vi "Write Contents.vi"(8 "Error in":errorcluster caption="Error in (no error)", 10 "Contents":refnum<class "Data Item.lvclass">[](array[class]), 11 "Element Array":refnum<class "Element Array.lvclass">) -> (0 "Error out":errorcluster, 3 "Element Array Out":refnum<class "Element Array.lvclass">)   [LabVIEW 2023, in "VILab.lvlib" / "Element Array.lvclass"]
uses:
  Element Array.lvclass
  Data Item.lvclass
  Attribute.lvclass/Attribute.ctl
  Element Array.lvclass/Element Array.ctl
  Attribute/Create Attribute (Data Item).vi
  Attribute.lvclass
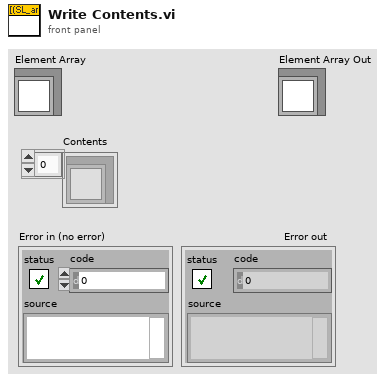
[diagram p1: front panel]
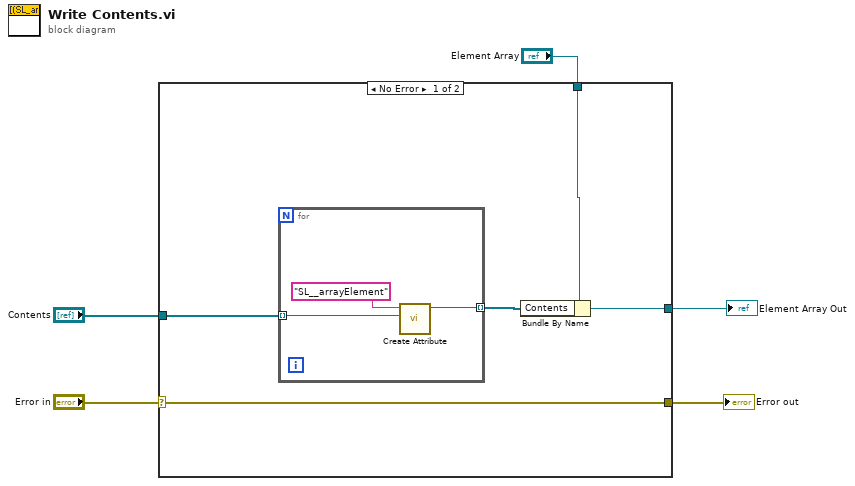
[diagram p0: block diagram]
diagram:
  n1 = case shown="No Error" "Error in" {
    selector: "Error in" -> [w7 w14]
    tunnel: "Contents" -> [w10 _]
    tunnel: [w8 w15] -> w4
    tunnel: [w7 w14] -> w3
    tunnel: "Element Array" -> [w6 w15]
    frame No Error {
      n2 = for {
        tunnel: w10 -> [w13] mode=indexing
        tunnel: [w11] -> w9 mode=indexing
        n3 = call-poly "Create Attribute.vi"("Value"=w13, "Name"="SL__arrayElement") -> ("Attribute"=w11:refnum<class "Attribute.lvclass">)  [unwired: 9 in]
      }
      n4 = Bundle By Name(cluster=w6, "Contents"=w9) -> (w8:refnum<class "Element Array.lvclass">)
    }
    frame Error {
    }
  }
  "Element Array Out" <- w4
  "Error out" <- w3
